vi "yaqc_get_turret_options.vi"(8 "error in (no error)":errorcluster, 9 "Yaqc Client In":refnum<k38>, 10 "Python Module Path In":path, 11 "Python Session In":refnum<k35>) -> (0 "error out":errorcluster, 1 "Yaqc Client Out":refnum<k38>, 2 "Python Module Path Out":path, 3 "Python Session Out":refnum<k35>, 4 "turret options":string[](array[string]))   [LabVIEW 2022 SP3]
doc: "Get current turret identifier."
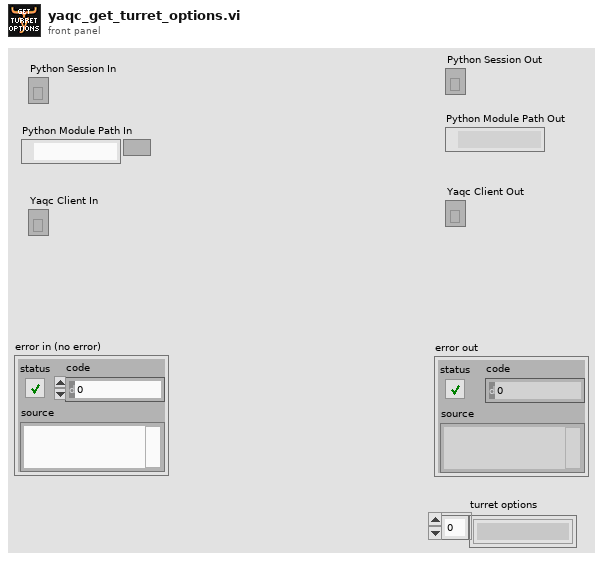
[diagram p1: front panel]
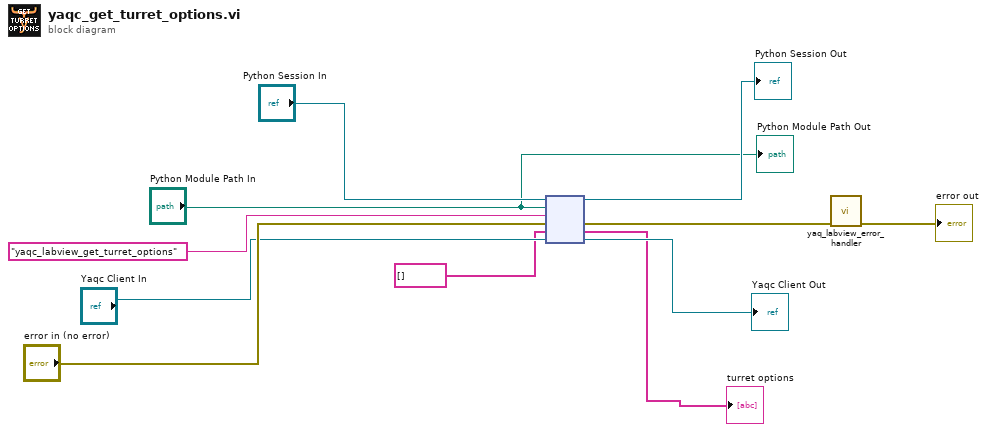
[diagram p0: block diagram]
diagram:
  n1 = node("Python Session In", "Python Module Path In", "yaqc_labview_get_turret_options" ("function name"), "error in (no error)", string[] [], "Yaqc Client In") -> (→"Python Session Out":refnum<k35>, w8:errorcluster, →"turret options":string[], →"Yaqc Client Out":refnum<k38>)  [unwired: 2 out]
  n2 = call "yaq_labview_error_handler.vi"("error in (no error)"=w8) -> ("error out"=→"error out":errorcluster)  [unwired: 10 in]
  "Python Module Path Out" <- "Python Module Path In"
